vi "Pfeiffer-RVC300.initialize interface.vi"(0 "i ref in":refnum<vi>, 1 "queryID":bool, 2 "resetDevice":bool, 3 "ms timeout (10000)":i32=10000, 5 "error in (no error)":errorcluster) -> (14 "i ref out":refnum<vi>, 15 "deviceID":string, 17 "timed out":bool, 19 "error out":errorcluster)   [LabVIEW 2014, in "Pfeiffer-RVC300.lvlib"]
doc: "Initializes the interface to the instrument. This method must be called prior to communicating with the instrument.\n\nLicense Agreement for this software:\n\nCopyright (C)\nMax-Planck-Institut für Kernphysik\nSaupfercheckweg 1\n69117 Heidelberg\nGermany\n\nContact: christopher.borgmann@mpi-hd.mpg.de\n\nThis program is free software: you can redistribute it and/or modify \nit under the terms of the GNU General Public License as published by\nthe Free Software Foundation, either version 3 of the License, or\n(at your option) any later version.\n\nThis program is distributed in the hope that it will be useful,\nbut WITHOUT ANY WARRANTY; without even the implied warranty of\nMERCHANTABILITY or FITNESS FOR A PARTICULAR PURPOSE. See the\nGNU General Public License for more details.\n\nYou should have received a copy of the GNU General Public License\nalong with this program. If not, see <http://www.gnu.org/licenses/>.\n\nMax-Planck-Institut für Kernphysik\nSaupfercheckweg 1, 69117 Heidelberg, Germany\nFor all questions and ideas contact: christopher.borgmann@mpi-hd.mpg.de\nLast update: 08.07.2010"
uses:
  Pfeiffer-RVC300.lvlib
  CS_Core/BaseProcess/BaseProcess.lvlib
  instr.lib/RVC300/RVC 300.lvlib
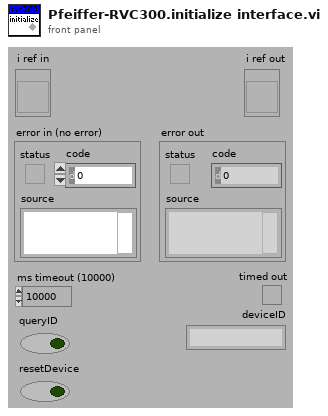
[diagram p1: front panel]
types:
  T1 = typedef "Pfeiffer-RVC300.lvlib/Pfeiffer-RVC300.i attribute.ctl" = cluster{"interfaceInitialized":bool, "VISAResource":refnum<visa-resource-name>, "WaitingTime":u32, "nomValues":T2, "actValues":T2}
  T2 = typedef "Pfeiffer-RVC300.lvlib/Pfeiffer-RVC300.parameters.ctl" = cluster{"regulationMode":T3, "valveType":string, "sensorType":string, "valveState":string, "flow":dbl, "pressure":dbl, "serviceIDs":cluster{"regulationModeID":i32, "valveTypeID":i32, "sensorTypeID":i32, "valveStateID":i32, "flowID":i32, "pressureID":i32}}
  T3 = typedef "Pfeiffer-RVC300.lvlib/Pfeiffer-RVC300.regulation mode.ctl" = enum16{"unknown", "Pressure", "Flow", "Wait"}
  T4 = typedef "BaseProcess.lvlib/BaseProcess.i attribute.ctl" = cluster{"EventStatus":string, "EventError":i32, "PresetEvtWatchD":i32, "PresetPdcWatchD":i32, "EventTimeout":i32, "PeriodicInterval":i32, "Interface":string[], "Address":string[], "Special":string[], "PeriodicError":i32, "PeriodicStatus":string, "SuperProc":string, "Descriptors":T5[], "CaseRef":refnum<vi>, "PdcRef":refnum<vi>, "Thread Ref":refnum<vi>, "eventErrorID":i32, "eventStatusID":i32, "periodicErrorID":i32, "periodicStatusID":i32, "pdcCtrID":i32}
  T5 = typedef "BaseProcess.lvlib/BaseProcess.descriptor definition.ctl" = cluster{"selector":string, "descriptor":T6}
  T6 = typedef "BaseProcess.lvlib/BaseProcess.descriptor string definition.ctl" = string
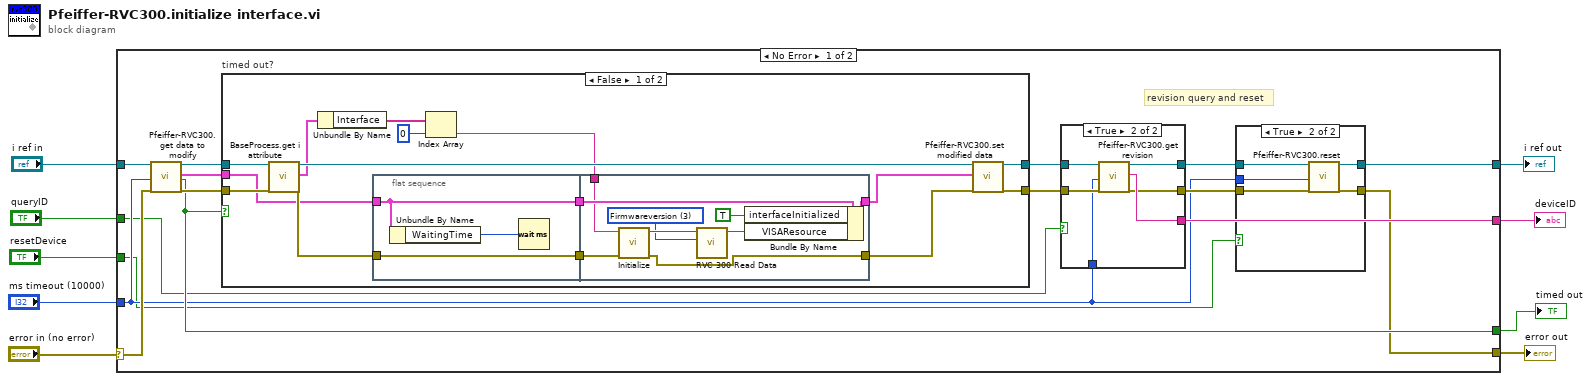
[diagram p0: block diagram]
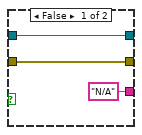
[diagram p3: hidden frame]
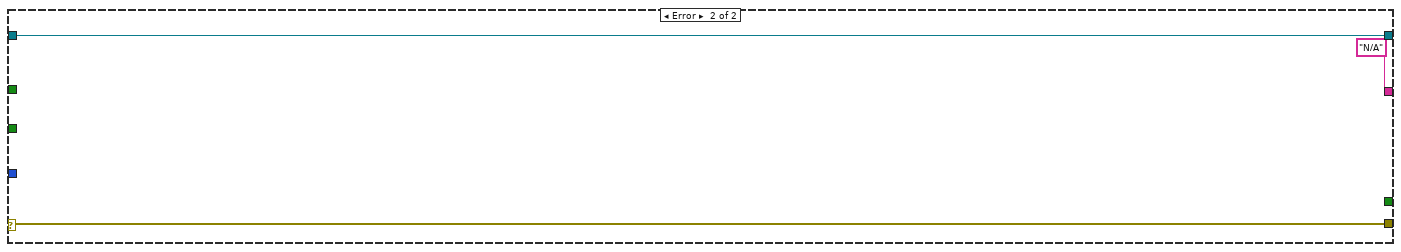
[diagram p5: hidden frame]
diagram:
  n1 = case shown="No Error" "error in (no error)" {
    selector: "error in (no error)" -> [w20 w72]
    tunnel: "i ref in" -> [w25 w73]
    tunnel: [w15 w73] -> w8
    tunnel: [w13 w72] -> w7
    tunnel: [w22 _] -> w6
    tunnel: "ms timeout (10000)" -> [w12 _]
    tunnel: [w19 "N/A" ("revision")] -> w3
    tunnel: "queryID" -> [w11 _]
    tunnel: "resetDevice" -> [w10 _]
    frame No Error {
      # "revision query and reset"
      n2 = call "Pfeiffer-RVC300.get data to modify.vi"("i ref in"=w25, "ms timeout (10000)"=w12, "error in (no error)"=w20) -> ("i ref out"=w24:refnum<vi>, "i attribute"=w21:T1, "timed out"=w22:bool, "error out"=w23:errorcluster)  [unwired: 13 in]
      n3 = case "timed out?" shown="False" w22 {
        tunnel: [w48 w70] -> w18
        tunnel: w24 -> [w55 w70]
        tunnel: [w47 w69] -> w17
        tunnel: w23 -> [w54 w69]
        tunnel: w21 -> [w45 _]
        frame False {
          n4 = call "BaseProcess.get i attribute.vi"("i ref in"=w55, "error in (no error)"=w54) -> ("i ref out"=w52:refnum<vi>, "i attribute"=w51:T4, "error out"=w53:errorcluster)  [unwired: 15 in]
          n5 = Unbundle By Name(w51) -> ("Interface"=w50:string[])
          n6 = flat-sequence {
            tunnel: w45 -> [w57]
            tunnel: w53 -> [w59]
            tunnel: [w59] -> w44
            tunnel: [w57] -> w43
            tunnel: [w68] -> w56
            tunnel: w42 -> [w60]
            tunnel: [w61] -> w46
            tunnel: w44 -> [w66]
            tunnel: w43 -> [w62]
            frame #0 {
              n7 = Unbundle By Name(w57) -> ("WaitingTime"=w58:u32)
              n8 = Wait (ms)(milliseconds to wait=w58) -> ()  [unwired: 1 out]
            }
            frame #1 {
              w64 = u16 3 items=["Mode", "Pressure", "Unit", "Firmwareversion", "Keyboard lock", "Pressure Setpoint", "Sensor Type", "Valve Type"] ("RVC 300 Read")
              n9 = call "Initialize.vi"("error in (no error)"=w66, "VISA resource name"=w60) -> ("error out"=w61:errorcluster, "duplicate VISA resource name"=w65:refnum<visa-resource-name>)  [unwired: 8 in]
              n10 = call "RVC 300 Read Data.vi"("RVC 300 Read"=w64, "Resource Name"=w65) -> ("Resource Name out"=w63:refnum<visa-resource-name>)  [unwired: 6 in, 3 out]
              n11 = Bundle By Name(cluster=w62, "interfaceInitialized"=TRUE, "VISAResource"=w63) -> (w68:T1)
            }
          }
          n12 = Index Array(array=w50, index=0) -> (element=w42:string)
          n13 = call "Pfeiffer-RVC300.set modified data.vi"("i ref in"=w52, "i attribute"=w56, "error in (no error)"=w46) -> ("i ref out"=w48:refnum<vi>, "error out"=w47:errorcluster)  [unwired: 15 in]
        }
        frame True {
        }
      }
      n14 = case shown="True" w11 {
        tunnel: ["N/A" ("revision") w41] -> w19
        tunnel: w18 -> [w35 w40]
        tunnel: w17 -> [w34 w39]
        tunnel: [w35 w38] -> w16
        tunnel: [w34 w37] -> w14
        tunnel: w12 -> [_ w36]
        frame False {
        }
        frame True {
          n15 = call "Pfeiffer-RVC300.get revision.vi"("i ref in"=w40, "ms timeout (10000)"=w36, "error in (no error)"=w39) -> ("i ref out"=w38:refnum<vi>, "revision"=w41:string, "error out"=w37:errorcluster)  [unwired: 13 in, 1 out]
        }
      }
      n16 = case shown="True" w10 {
        tunnel: w16 -> [w27 w32]
        tunnel: [w27 w31] -> w15
        tunnel: w14 -> [w26 w30]
        tunnel: [w26 w29] -> w13
        tunnel: w12 -> [_ w28]
        frame False {
        }
        frame True {
          n17 = call "Pfeiffer-RVC300.reset.vi"("i ref in"=w32, "ms timeout (10000)"=w28, "error in (no error)"=w30) -> ("i ref out"=w31:refnum<vi>, "error out"=w29:errorcluster)  [unwired: 15 in]
        }
      }
    }
    frame Error {
    }
  }
  "error out" <- w7
  "i ref out" <- w8
  "timed out" <- w6
  "deviceID" <- w3
